vi "Create Linked List.vi"(8 "error in (no error)":errorcluster, 11 "Linked List in":refnum<class "Linked List.lvclass">) -> (0 "error out":errorcluster, 3 "Linked List out":refnum<class "Linked List.lvclass">)   [LabVIEW 2020, in "Linked Lists.lvlib" / "Linked List.lvclass"]
uses:
  <vilib>/gpm_packages/@cs/linked-list/Source/Linked List/Linked List/Linked List.lvclass
  <vilib>/gpm_packages/@cs/linked-list/Source/Linked List/Linked List/Linked List.lvclass/Linked List.ctl
  <vilib>/gpm_packages/@cs/lookup-table/Source/LookupTable/LookupTable.lvclass
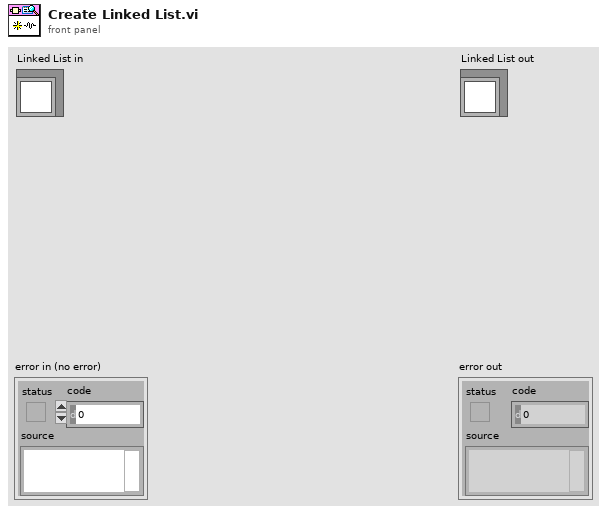
[diagram p1: front panel]
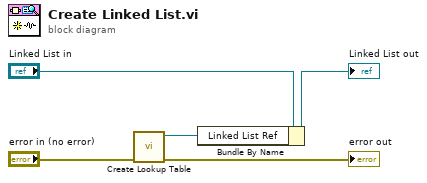
[diagram p0: block diagram]
diagram:
  n1 = call <vilib>:"Create Lookup Table.vi"("error in (no error)"="error in (no error)") -> ("error out"=→"error out":errorcluster, "LookupTable Reference"=w1:refnum<data-value>)  [unwired: 9 in]
  n2 = Bundle By Name(cluster="Linked List in", "Linked List Ref"=w1) -> (→"Linked List out":refnum<class "Linked List.lvclass">)
